vi "Acquire_wp_nodt.vi"(0 "Ch Armed Reg":refnum<k21>="Register 1", 1 "Command FIFO":refnum<k21>, 3 "Circular Buffer Mem":refnum<k21>, 4 "circular buffer length":u32=300, 5 "FPGA I/O In":refnum<k21>="IO Module\\AI A0", 7 "channel on/off":bool, 9 "Trigger":i16=1500, 10 "Timing FIFO":refnum<k21>, 11 "Samples to Acquire":u32=100, 12 "Simulate":bool, 13 "Is Test Pulse?":bool, 14 "# of pretrigger":u32=15, 15 "timing":u64) -> ()   [LabVIEW 2012]
uses:
  <vilib>/rvi/DataTransferAndStorage/Container/Common/niFpgaContainerExecOnDevCompGetState.vi
  <vilib>/rvi/Memory/Memory_Emulation/nirvimemoryEmulationManagerCache_GetValue.vi
  <vilib>/rvi/Memory/Memory_Emulation/niFpgaMemoryEmulationValidateCache.vi
  <vilib>/rvi/DataTransferAndStorage/Container/Common/niFpgaContainerGetUniqueNameForEmu.vi
  <vilib>/rvi/Memory/Memory_Emulation/nirvimemoryEmulationManagerCache_InsertValue.vi
  <vilib>/rvi/eio/common/nirviEmuTemplateMethod_errors.vi
  <vilib>/rvi/Emulation/niFpgaSctlEmulationGetInTimedLoop.vi
  <vilib>/rvi/FIFO/Fifo_Resource/nirvififoEmulationSetSize.vi
  <vilib>/rvi/errors/niFpgaSetErrorForExecOnDevCompSimple.vi
  <vilib>/rvi/eio/common/nirviEmuReportErrorAndStop.vi
  <vilib>/rvi/Emulation/niFpgaSctlEmulationFifoFullMgr.vi
  <vilib>/rvi/Emulation/niFpgaSctlEmulationResourceMgr.vi
  <vilib>/rvi/interface/RandomDataEmulation/nirviRandomDataFPGAFIFO.vi
  <vilib>/rvi/interface/RandomDataEmulation/niFpgaRandomDataHandleErrors.vi
  <vilib>/rvi/DataTransferAndStorage/Container/XNode/niFpgaContainer.xnode
  <vilib>/rvi/DataTransferAndStorage/Register/Emulation/niFpgaRegisterEmulationRefIn.vi
  <vilib>/eio/EIONode/EIONode.xnode
  <vilib>/rvi/FIFO/Fifo_Resource/niFpgaFifoEmulationRefIn.vi
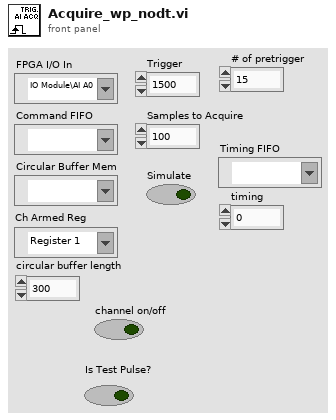
[diagram p1: front panel]
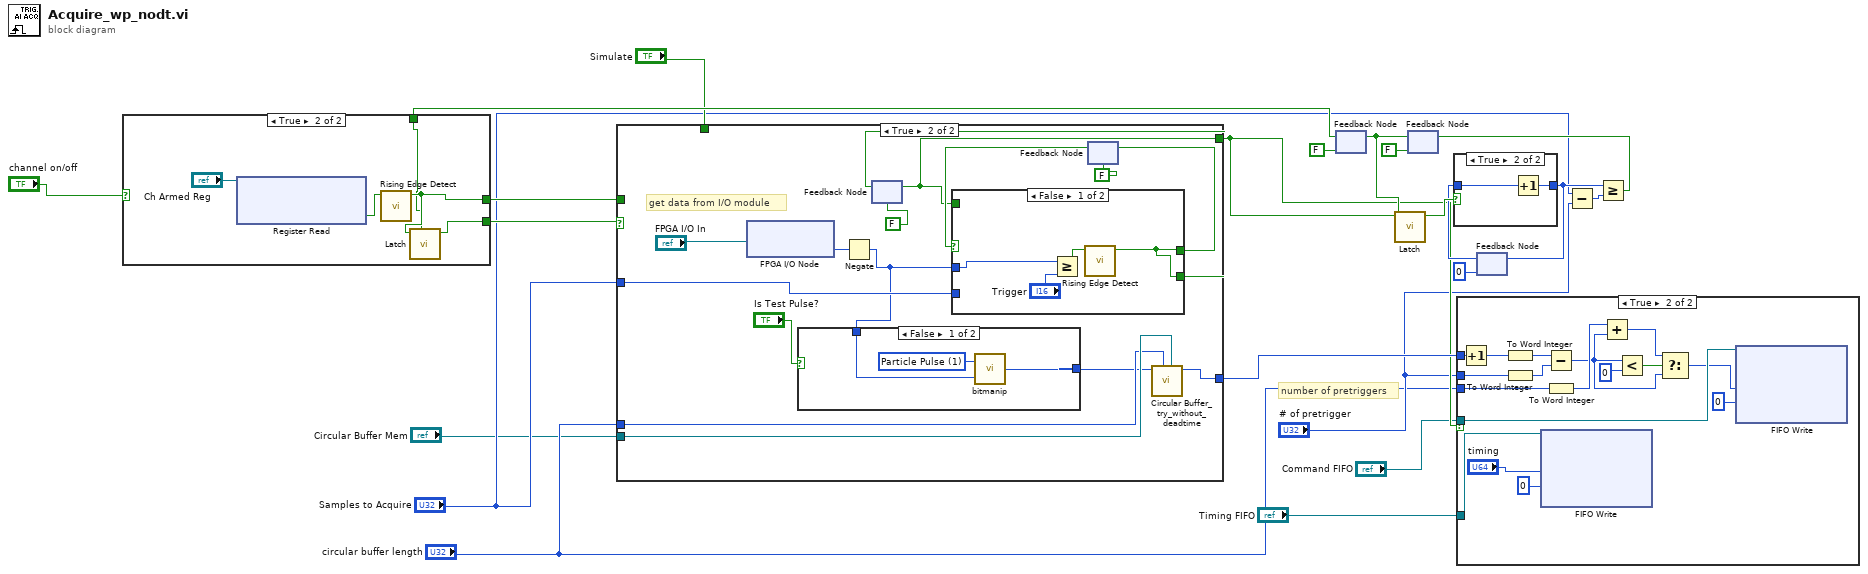
[diagram p0: block diagram]
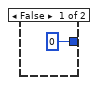
[diagram p3: hidden frame]
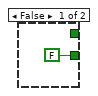
[diagram p4: hidden frame]
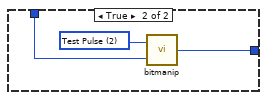
[diagram p6: hidden frame]
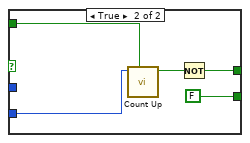
[diagram p7: hidden frame]
diagram:
  # "number of pretriggers"
  n1 = feedback #1(FALSE) -> (w17:bool)
  n2 = case shown="True" "channel on/off" {
    tunnel: [FALSE ("Output") w27] -> w22
    tunnel: [_ w28] -> w21
    tunnel: w17 -> [_ w26]
    frame False {
    }
    frame True {
      n3 = xnode ("Register Read")("Register In"="Ch Armed Reg") -> ("Data"=w24:bool)  [unwired: 1 out]
      n4 = call "Rising Edge Detect.vi"("Input"=w24) -> ("Rising Edge"=w28:bool)  [unwired: 10 in]
      n5 = call "Latch.vi"("Reset"=w26, "Input"=w28) -> ("Output"=w27:bool)  [unwired: 9 in]
    }
  }
  n6 = case shown="True" w22 {
    tunnel: "Circular Buffer Mem" -> [_ w43]
    tunnel: "circular buffer length" -> [_ w38]
    tunnel: [_ w42] -> w20
    tunnel: w21 -> [_ _]
    tunnel: "Samples to Acquire" -> [_ w37]
    tunnel: "Simulate" -> [_ _]
    tunnel: [_ w33] -> w9
    frame False {
    }
    frame True {
      # "get data from I/O module"
      n7 = xnode "FPGA I/O Node"("FPGA I/O In"="FPGA I/O In") -> ("I/O Item"=w41:i16)  [unwired: 1 out]
      n8 = Negate(x=w41) -> (-x=w31:i16)
      n9 = case shown="False" "Is Test Pulse?" {
        tunnel: w31 -> [w45 w48]
        tunnel: [w44 w47] -> w30
        frame False {
          w46 = u16 1 items=["Header Information", "Particle Pulse", "Test Pulse"] ("Pulse Type")
          n10 = call "bitmanip.vi"("Pulse Type"=w46, "Integer to be written"=w45) -> ("Integer Written"=w44:i16)  [unwired: 2 in]
        }
        frame True {
          w49 = u16 2 items=["Header Information", "Particle Pulse", "Test Pulse"] ("Pulse Type")
          n11 = call "bitmanip.vi"("Pulse Type"=w49, "Integer to be written"=w48) -> ("Integer Written"=w47:i16)  [unwired: 2 in]
        }
      }
      n12 = feedback #2(FALSE) -> (w33:bool)
      n13 = feedback #3(FALSE) -> (w36:bool)
      n14 = case shown="False" w36 {
        tunnel: w31 -> [w53 _]
        tunnel: w37 -> [_ w58]
        tunnel: w33 -> [_ w57]
        tunnel: [w51 w55] -> w35
        tunnel: [w51 FALSE] -> w34
        frame False {
          n15 = Greater Or Equal?(x=w53, y="Trigger") -> (x >= y?=w52:bool)
          n16 = call "Rising Edge Detect.vi"("Input"=w52) -> ("Rising Edge"=w51:bool)  [unwired: 10 in]
        }
        frame True {
          n17 = call "Count Up.vi"("Reset?"=w57, "goal"=w58) -> ("Count Met"=w56:bool)  [unwired: 8 in, 1 out]
          n18 = Not(x=w56) -> (.not. x?=w55:bool)
        }
      }
      n19 = feedback-in #2(w34) -> ()
      n20 = feedback-in #3(w35) -> ()
      n21 = call "Circular Buffer_try_without_deadtime.vi"("Refnum in"=w43, "circular buffer length"=w38, "Data"=w30) -> ("Address"=w42:u16)  [unwired: 8 in]
    }
  }
  n22 = feedback #4(FALSE) -> (w15:bool)
  n23 = feedback-in #1(w15) -> ()
  n24 = call "Latch.vi"("Reset"=w15, "Input"=w9) -> ("Output"=w13:bool)  [unwired: 9 in]
  n25 = case shown="True" w9 {
    tunnel: "Command FIFO" -> [_ w75]
    tunnel: "Timing FIFO" -> [_ w74]
    tunnel: w20 -> [_ w63]
    tunnel: "circular buffer length" -> [_ w61]
    tunnel: "# of pretrigger" -> [_ w60]
    frame False {
    }
    frame True {
      n26 = Increment(x=w63) -> (x+1=w69:u16)
      n27 = To Word Integer(number=w69) -> (16bit integer=w70:i16)
      n28 = To Word Integer(number=w60) -> (16bit integer=w71:i16)
      n29 = xnode ("FIFO Write")("Element"="timing", "Timeout"=0, "FIFO In"=w74) -> ()  [unwired: 2 out]
      n30 = Subtract(x=w70, y=w71) -> (x-y=w67:i16)
      n31 = To Word Integer(number=w61) -> (16bit integer=w68:i16)
      n32 = Add(x=w68, y=w67) -> (x+y=w66:i16)
      n33 = Less?(x=w67, y=i16 0) -> (x < y?=w64:bool)
      n34 = Select(t=w66, s=w64, f=w67) -> (s? t:f=w62:i16)
      n35 = xnode ("FIFO Write")("Element"=w62, "Timeout"=0, "FIFO In"=w75) -> ()  [unwired: 2 out]
    }
  }
  n36 = feedback #5(u32 0) -> (w12:u32)
  n37 = case shown="True" w13 {
    tunnel: w12 -> [_ w78]
    tunnel: [i16 0 w77] -> w10
    frame False {
    }
    frame True {
      n38 = Increment(x=w78) -> (x+1=w77:u32)
    }
  }
  n39 = feedback-in #5(w10) -> ()
  n40 = Subtract(x="Samples to Acquire", y="# of pretrigger") -> (x-y=w11:u32)
  n41 = Greater Or Equal?(x=w10, y=w11) -> (x >= y?=w16:bool)
  n42 = feedback-in #4(w16) -> ()
